vi "Slave.vi"() -> ()   [LabVIEW 2018]
panel:
  out "时间戳":u64 format="%016x"
  out "帧号":u16 format="%04x"
  in  "从站IP":string="192.168.3.100"
  in  "停止":bool
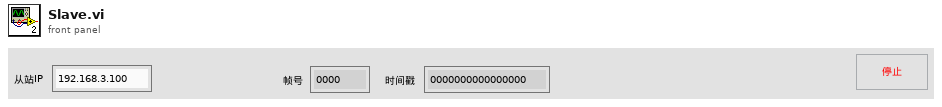
[diagram p1: front panel]
types:
  T1 = cluster{"主站IP":u32, "组号":u8, "帧号":u16, "时间戳":u64}
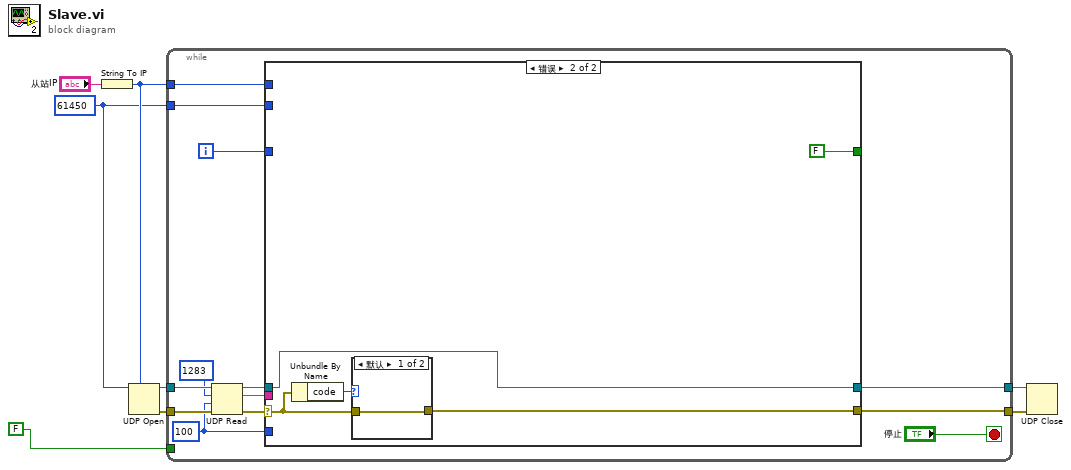
[diagram p0: block diagram]
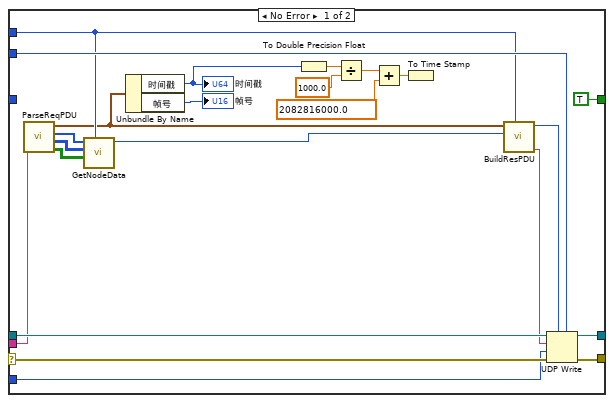
[diagram p2: hidden frame]
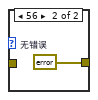
[diagram p3: hidden frame]
diagram:
  w2 = u16 61450 ("端口")
  n1 = String To IP(1:"从站IP") -> (0:w3:u32)
  n2 = UDP Open(7:w3, 11:w2) -> (port=w8:refnum<k16>, 0:w6:errorcluster)  [unwired: 3 in, 1 out]
  n3 = while {
    tunnel: w8 -> [w21]
    tunnel: [w12] -> w7
    tunnel: w6 -> [w20]
    tunnel: [w17] -> w5
    tunnel: w3 -> [w14]
    tunnel: w2 -> [w13]
    tunnel: FALSE -> [_]
    i -> [w10]
    stop <- "停止" stop-if-true
    w11 = 100 ("超时毫秒(25000)")
    n4 = UDP Read(connection ID=w21, max size (548)=1283 ("最大值(548)"), timeout ms (25000)=w11, 8:w20) -> (data out=w18:string, error out=w19:errorcluster, 3:w15:refnum<k16>)  [unwired: 2 out]
    n5 = case shown="错误" w19 {
      selector: w19 -> [w43 w48]
      tunnel: w18 -> [w38 _]
      tunnel: [w42 w47] -> w17
      tunnel: [TRUE FALSE] -> _
      tunnel: w15 -> [w41 w45]
      tunnel: w14 -> [w35 _]
      tunnel: w13 -> [w39 _]
      tunnel: [w40 w45] -> w12
      tunnel: w11 -> [w30 _]
      tunnel: w10 -> [_ _]
      frame No Error {
        n6 = call "ParseReqPDU.vi"("数据in"=w38) -> ("All RY"=w31:bool[][], "All RWw"=w32:u16[][], "从站IP组"=w34:u32[], "主站信息"=w29:T1)  [unwired: 7 in]
        n7 = call "GetNodeData.vi"("指定从站IP"=w35, "All RY in"=w31, "All RWw in"=w32, "从站IP组"=w34) -> ("占用站数"=w33:i32)  [unwired: 5 in, 2 out]
        n8 = Unbundle By Name(w29) -> ("时间戳"=w24:u64, "帧号"=→"帧号":u16)
        "时间戳" <- w24
        n9 = To Double Precision Float(number=w24) -> (double precision float=w28:dbl)
        n10 = Divide(x=w28, y=1000.0) -> (x/y=w26:dbl)
        n11 = Add(x=w26, y=2082816000.0 ("双精度浮点数")) -> (x+y=w22:dbl)
        n12 = To Time Stamp(1:w22) -> ()  [unwired: 1 out]
        n13 = call "BuildResPDU.vi"("从站IP"=w35, "占用站数"=w33, "主站信息"=w29) -> ("输出字符串"=w37:string, "主站IP"=w36:u32)  [unwired: 7 in]
        n14 = UDP Write(address=w36, port or service name=w39, connection ID=w41, data in=w37, 8:w43, 9:w30) -> (error out=w42:errorcluster, 3:w40:refnum<k16>)
      }
      frame Error {
        n15 = Unbundle By Name(w48) -> ("code"=w49:i32)
        n16 = case shown="默认" w49 {
          tunnel: [w50 w51] -> w47
          tunnel: w48 -> [w50 _]
          frame Default {
          }
          frame 56 {
            w51 = errorcluster {"status"=FALSE, "code"=0, "source"=""}  # 无错误
          }
        }
      }
    }
  }
  n17 = UDP Close(connection ID=w7, 8:w5) -> ()  [unwired: 2 out]
